vi "Teleop.vi"(10 "Match Info":T1={"Autonomous Elapsed Seconds"=0.0, "TeleOp Elapsed Seconds"=0.0, "Disabled Elapsed Seconds"=0.0, "Visited Autonomous"=FALSE, "Visited TeleOp"=FALSE, "Visited Disabled"=FALSE, "Autonomous Settings"={"Autonomous Style"=enum."Independent", "VI Refnum"=refnum}}, 11 "Call Context":T2) -> ()   [LabVIEW 2017]
doc: "This VI is called for each TeleOp packet received from the DS where the robot is not disabled. It is often used to read from the joysticks and update I/O or to update setpoints for timed control loops. It should complete and return within 20 milliseconds or it may miss DS packets."
uses:
  <vilib>/Rock Robotics/WPI/DriverStation/WPI_DriverStationDerivedRobotMode.ctl
  <vilib>/Rock Robotics/WPI/DriverStation/WPI_DriverStationMatch Info.ctl
  <vilib>/Rock Robotics/WPI/Utilities/WPI_GetSetVariantRefNum.vi
  <vilib>/Rock Robotics/Network Tables/NT Write Boolean Array.vi
  <vilib>/Rock Robotics/Network Tables/NT Write Numeric Array.vi
  <vilib>/Rock Robotics/Network Tables/NT Read Boolean.vi
  <vilib>/Rock Robotics/Network Tables/NT Read Number.vi
  <vilib>/Rock Robotics/WPI/RobotDrive/WPI_RobotDriveMecanumDrive_Cartesian.vi
panel:
  out "Numeric":dbl
  out "Sample Slider 0":dbl(slide) scale=0.0..5.0
  out "Sample Boolean 1":bool
  out "Sample Boolean 0":bool
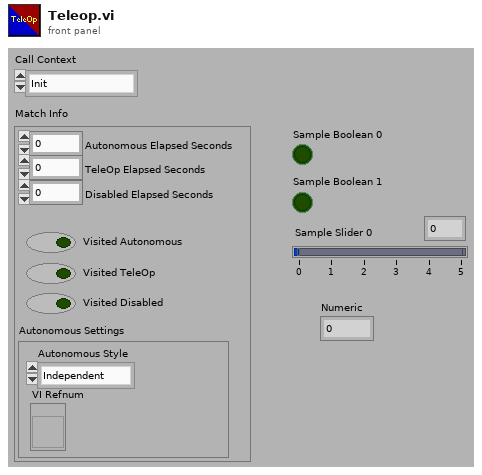
[diagram p1: front panel]
types:
  T1 = typedef "WPI_DriverStationMatch Info.ctl" = cluster{"Autonomous Elapsed Seconds":dbl, "TeleOp Elapsed Seconds":dbl, "Disabled Elapsed Seconds":dbl, "Visited Autonomous":bool, "Visited TeleOp":bool, "Visited Disabled":bool, "Autonomous Settings":cluster{"Autonomous Style":enum16{"Iterative", "Independent"}, "VI Refnum":refnum<vi>}}
  T2 = typedef "WPI_DriverStationDerivedRobotMode.ctl" = enum16{"Init", "Execute", "Stop"}
  T3 = typedef "WPI_JoystickDevRef.ctl" = cluster{"Device":T4}
  T4 = typedef "WPI_JoystickDeviceEnum.ctl" = enum16{"USB 0", "USB 1", "USB 2", "USB 3", "USB 4", "USB 5"}
  T5 = typedef "WPI_MotorControlDeviceRef.ctl" = cluster{"DeviceStatus":errorcluster, "Type":T6, "PWM":cluster{"PWM Channel":T7, "DeadBand":T8}, "CAN":cluster{"Device Number":u8, "SetOutput VI Ref":variant, "GetOutput VI Ref":variant, "Enable VI Ref":variant, "Disable VI Ref":variant, "Data":variant}, "Invert":bool, "DIO PWM":cluster{"PWM \"Enable\" Channel":T7, "DIOChannel":T9, "PWM Rate":dbl}}
  T6 = typedef "WPI_MotorControlType.ctl" = enum16{"PWM", "CAN", "DIO PWM"}
  T7 = typedef "FPGA_DIOPWMChannel.ctl" = enum8{"PWM 0", "PWM 1", "PWM 2", "PWM 3", "PWM 4", "PWM 5", "PWM 6", "PWM 7", "PWM 8", "PWM 9", "PWM MXP 0", "PWM MXP 1", "PWM MXP 2", "PWM MXP 3", "PWM MXP 4", "PWM MXP 5", "PWM MXP 6", "PWM MXP 7", "PWM MXP 8", "PWM MXP 9", "Invalid"}
  T8 = typedef "WPI_PWMDeadband.ctl" = cluster{"Name":string, "maxPositivePwm":i32, "minPositivePwm":i32, "centerPwm":i32, "maxNegativePwm":i32, "minNegativePwm":i32, "angularRange":u16}
  T9 = typedef "FPGA_DIOChannel.ctl" = enum8{"DIO 0", "DIO 1", "DIO 2", "DIO 3", "DIO 4", "DIO 5", "DIO 6", "DIO 7", "DIO 8", "DIO 9", "DIO MXP 0", "DIO MXP 1", "DIO MXP 2", "DIO MXP 3", "DIO MXP 4", "DIO MXP 5", "DIO MXP 6", "DIO MXP 7", "DIO MXP 8", "DIO MXP 9", "DIO MXP 10", "DIO MXP 11", "DIO MXP 12", "DIO MXP 13", "DIO MXP 14", "DIO MXP 15", "SPI Port CS1", "SPI Port CS2", "SPI Port CS3", "SPI Port MISO", "SPI Port MOSI", "Invalid"}
  T10 = typedef "WPI_RobotDriveDevRef.ctl" = cluster{"DevStatus":errorcluster, "Motors[]":T5[], "Square Inputs":bool, "Max Output":dbl}
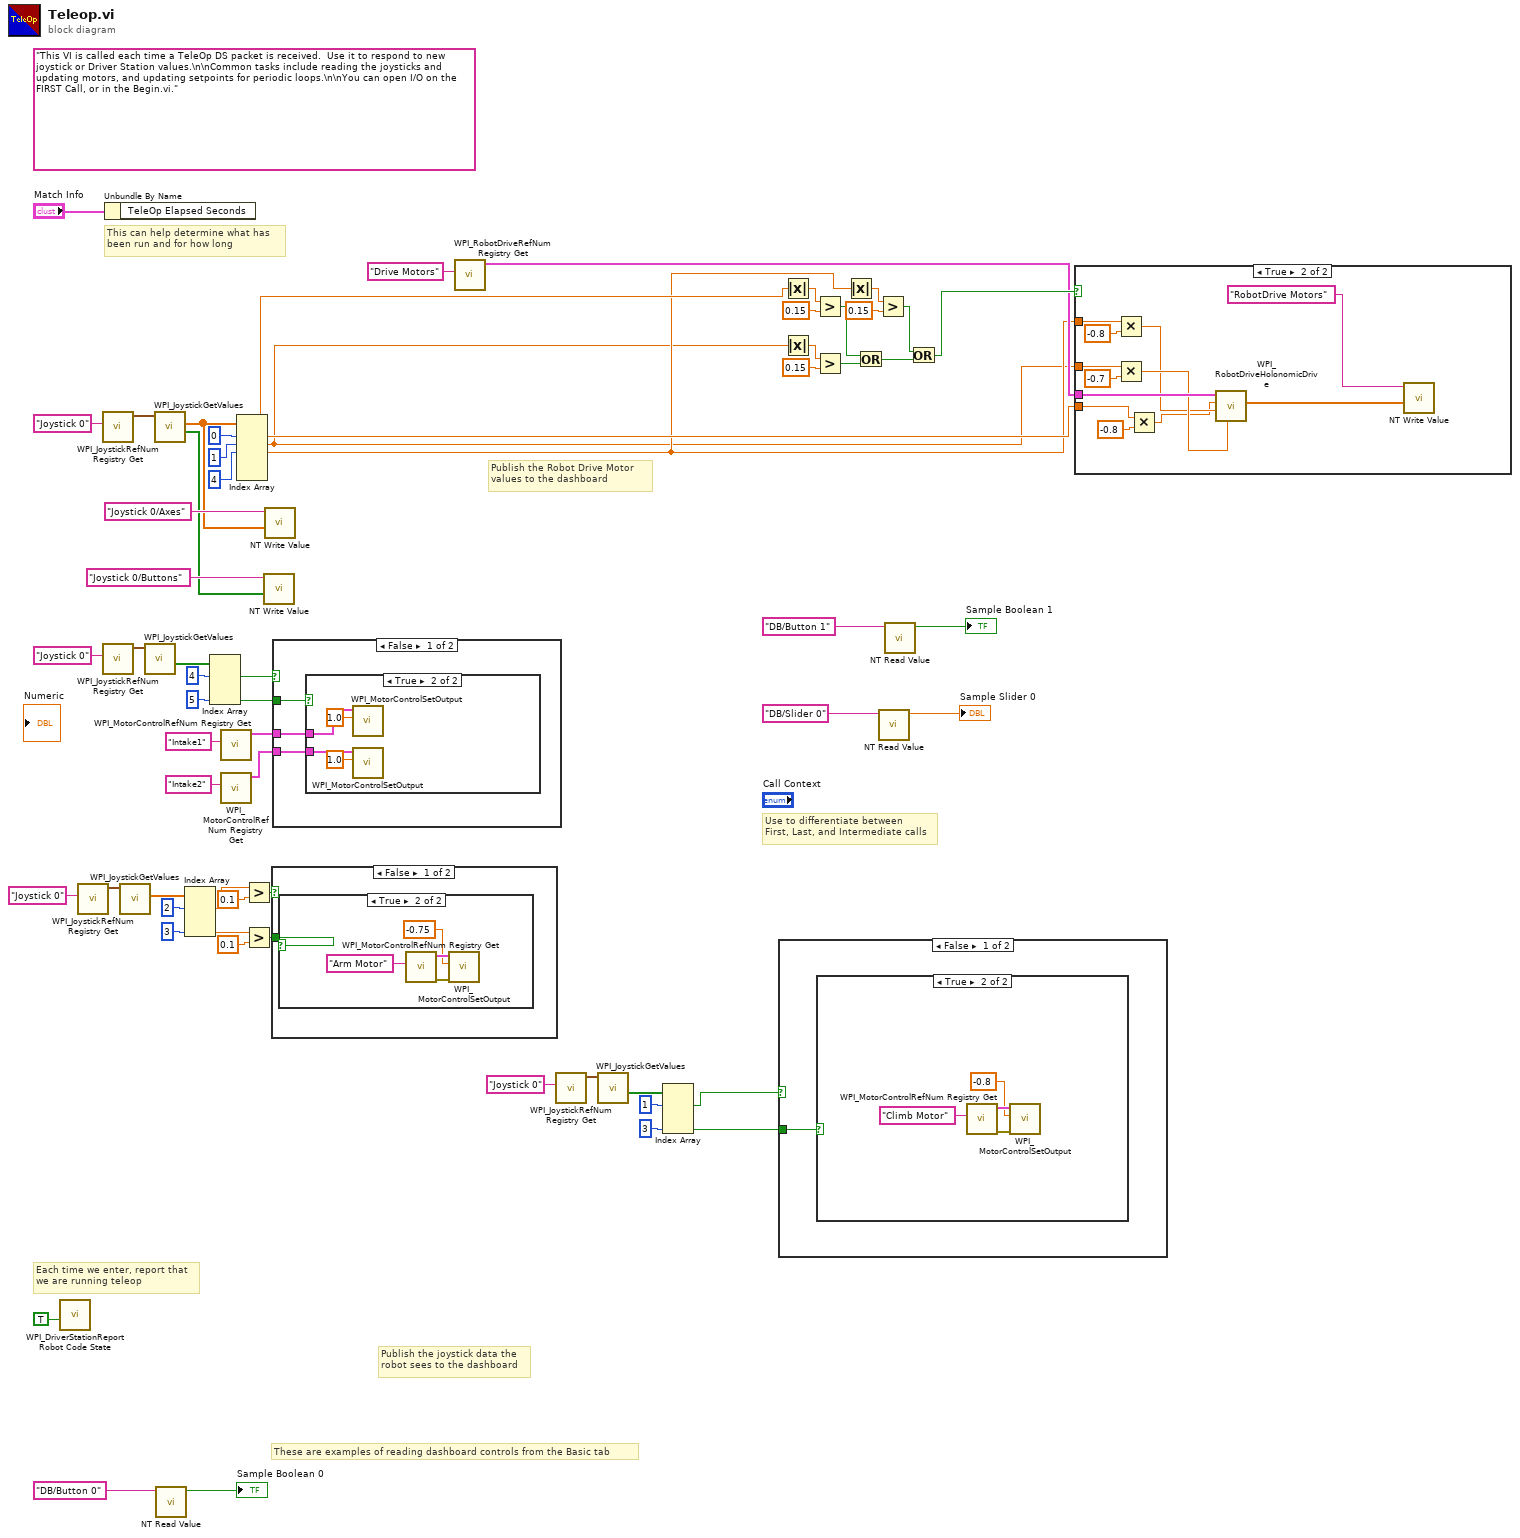
[diagram p0: block diagram]
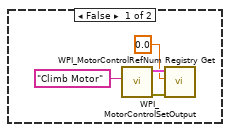
[diagram p3: hidden frame]
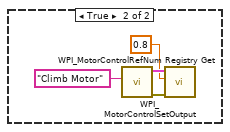
[diagram p4: hidden frame]
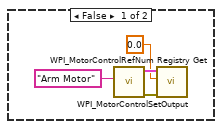
[diagram p5: hidden frame]
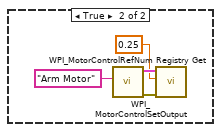
[diagram p6: hidden frame]
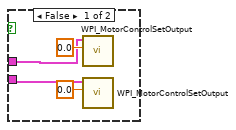
[diagram p7: hidden frame]
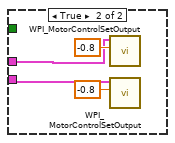
[diagram p8: hidden frame]
diagram:
  (unwired) "This VI is called each time a TeleOp DS packet is received.  Use it to respond to new joystick or Driver Station values.\n\nCommon tasks include reading the joysticks and updating motors, and updating setpoints for periodic loops.\n\nYou can open I/O on the FIRST Call, or in the Begin.vi."
  # "These are examples of reading dashboard controls from the Basic tab"
  # "Publish the Robot Drive Motor\nvalues to the dashboard"
  # "Publish the joystick data the\nrobot sees to the dashboard"
  # "Each time we enter, report that\nwe are running teleop"
  # "Use to differentiate between\nFirst, Last, and Intermediate calls"
  # "This can help determine what has\nbeen run and for how long"
  n1 = call <vilib>:"WPI_DriverStationReport Robot Code State.vi"("TeleOp"=TRUE ("Autonomous")) -> ()  [unwired: 10 in, 1 out]
  n2 = call <vilib>:"WPI_JoystickRefNum Registry Get.vi"("refnum name"="Joystick 0") -> ("JoystickDevRef"=w36:T3)  [unwired: 1 in, 9 out]
  n3 = call <vilib>:"WPI_JoystickRefNum Registry Get.vi"("refnum name"="Joystick 0") -> ("JoystickDevRef"=w59:T3)  [unwired: 1 in, 9 out]
  n4 = call <vilib>:"WPI_JoystickRefNum Registry Get.vi"("refnum name"="Joystick 0") -> ("JoystickDevRef"=w46:T3)  [unwired: 1 in, 9 out]
  n5 = Unbundle By Name("Match Info") -> ()  [unwired: 1 out]
  n6 = call <vilib>:"WPI_JoystickGetValues.vi"("JoystickDevRef"=w36) -> ("Axes"=w33:dbl[])  [unwired: 6 in, 4 out]
  n7 = call <vilib>:"WPI_JoystickGetValues.vi"("JoystickDevRef"=w46) -> ("Buttons"=w40:bool[])  [unwired: 6 in, 4 out]
  n8 = call <vilib>:"WPI_JoystickGetValues.vi"("JoystickDevRef"=w59) -> ("Buttons"=w54:bool[], "Axes"=w55:dbl[])  [unwired: 6 in, 3 out]
  n9 = call-poly <vilib>:"NT Read Value.vi"("Name"="DB/Button 0" ("refnum name")) -> ("Boolean"=→"Sample Boolean 0":bool)  [unwired: 9 in, 1 out]
  n10 = Index Array(array=w33, index #1=2 ("index"), index #4=3 ("index")) -> (element #1=w32:dbl, element #4=w29:dbl)  [unwired: 2 in, 2 out]
  n11 = Index Array(array=w40, index #1=4 ("index"), index #4=5 ("index")) -> (element #1=w39:bool, element #4=w38:bool)  [unwired: 2 in, 2 out]
  n12 = call <vilib>:"WPI_MotorControlRefNum Registry Get.vi"("refnum name"="Intake1") -> ("MotorControlDevRef"=w1:T5)  [unwired: 9 in, 1 out]
  n13 = call <vilib>:"WPI_MotorControlRefNum Registry Get.vi"("refnum name"="Intake2") -> ("MotorControlDevRef"=w2:T5)  [unwired: 9 in, 1 out]
  n14 = Index Array(array=w55, index #1=0 ("index"), index #2=1 ("index"), index #3=4 ("index")) -> (element #1=w10:dbl, element #2=w6:dbl, element #3=w8:dbl)  [unwired: 3 in, 3 out]
  n15 = Greater?(x=w32, y=0.1) -> (0:w30:bool)
  n16 = Greater?(x=w29, y=0.1) -> (0:w20:bool)
  n17 = call-poly <vilib>:"NT Write Value.vi"("Boolean Array"=w54, "Name"="Joystick 0/Buttons") -> ()  [unwired: 9 in, 1 out]
  n18 = call-poly <vilib>:"NT Write Value.vi"("Numeric Array"=w55, "Name"="Joystick 0/Axes") -> ()  [unwired: 9 in, 1 out]
  n19 = case shown="False" w30 {
    tunnel: w20 -> [w63 _]
    frame False {
      n20 = case shown="True" w63 {
        frame False {
          n21 = call <vilib>:"WPI_MotorControlRefNum Registry Get.vi"("refnum name"="Arm Motor") -> ("error out"=w67:errorcluster, "MotorControlDevRef"=w66:T5)  [unwired: 9 in]
          n22 = call <vilib>:"WPI_MotorControlSetOutput.vi"("error in (no error)"=w67, "Output"=0.0, "MotorControlDevRef"=w66) -> ()  [unwired: 6 in, 3 out]
        }
        frame True {
          n23 = call <vilib>:"WPI_MotorControlRefNum Registry Get.vi"("refnum name"="Arm Motor") -> ("error out"=w71:errorcluster, "MotorControlDevRef"=w70:T5)  [unwired: 9 in]
          n24 = call <vilib>:"WPI_MotorControlSetOutput.vi"("error in (no error)"=w71, "Output"=-0.75, "MotorControlDevRef"=w70) -> ()  [unwired: 6 in, 3 out]
        }
      }
    }
    frame True {
      n25 = call <vilib>:"WPI_MotorControlRefNum Registry Get.vi"("refnum name"="Arm Motor") -> ("error out"=w75:errorcluster, "MotorControlDevRef"=w74:T5)  [unwired: 9 in]
      n26 = call <vilib>:"WPI_MotorControlSetOutput.vi"("error in (no error)"=w75, "Output"=0.25, "MotorControlDevRef"=w74) -> ()  [unwired: 6 in, 3 out]
    }
  }
  n27 = case shown="False" w39 {
    tunnel: w38 -> [w78 _]
    tunnel: w2 -> [w77 w87]
    tunnel: w1 -> [w76 w88]
    frame False {
      n28 = case shown="True" w78 {
        tunnel: w77 -> [w79 w86]
        tunnel: w76 -> [w80 w85]
        frame False {
          n29 = call <vilib>:"WPI_MotorControlSetOutput.vi"("Output"=0.0, "MotorControlDevRef"=w80) -> ()  [unwired: 7 in, 3 out]
          n30 = call <vilib>:"WPI_MotorControlSetOutput.vi"("Output"=0.0, "MotorControlDevRef"=w79) -> ()  [unwired: 7 in, 3 out]
        }
        frame True {
          n31 = call <vilib>:"WPI_MotorControlSetOutput.vi"("Output"=1.0, "MotorControlDevRef"=w85) -> ()  [unwired: 7 in, 3 out]
          n32 = call <vilib>:"WPI_MotorControlSetOutput.vi"("Output"=1.0, "MotorControlDevRef"=w86) -> ()  [unwired: 7 in, 3 out]
        }
      }
    }
    frame True {
      n33 = call <vilib>:"WPI_MotorControlSetOutput.vi"("Output"=-0.8, "MotorControlDevRef"=w88) -> ()  [unwired: 7 in, 3 out]
      n34 = call <vilib>:"WPI_MotorControlSetOutput.vi"("Output"=-0.8, "MotorControlDevRef"=w87) -> ()  [unwired: 7 in, 3 out]
    }
  }
  n35 = call <vilib>:"WPI_RobotDriveRefNum Registry Get.vi"("refnum name"="Drive Motors") -> ("RobotDriveDevRef"=w11:T10)  [unwired: 1 in, 9 out]
  n36 = call <vilib>:"WPI_JoystickRefNum Registry Get.vi"("refnum name"="Joystick 0") -> ("JoystickDevRef"=w26:T3)  [unwired: 1 in, 9 out]
  n37 = call <vilib>:"WPI_JoystickGetValues.vi"("JoystickDevRef"=w26) -> ("Buttons"=w23:bool[])  [unwired: 6 in, 4 out]
  n38 = Index Array(array=w23, index #1=1 ("index"), index #4=3 ("index")) -> (element #1=w22:bool, element #4=w21:bool)  [unwired: 2 in, 2 out]
  n39 = case shown="False" w22 {
    tunnel: w21 -> [w91 _]
    frame False {
      n40 = case shown="True" w91 {
        frame False {
          n41 = call <vilib>:"WPI_MotorControlRefNum Registry Get.vi"("refnum name"="Climb Motor") -> ("error out"=w95:errorcluster, "MotorControlDevRef"=w94:T5)  [unwired: 9 in]
          n42 = call <vilib>:"WPI_MotorControlSetOutput.vi"("error in (no error)"=w95, "Output"=0.0, "MotorControlDevRef"=w94) -> ()  [unwired: 6 in, 3 out]
        }
        frame True {
          n43 = call <vilib>:"WPI_MotorControlRefNum Registry Get.vi"("refnum name"="Climb Motor") -> ("error out"=w99:errorcluster, "MotorControlDevRef"=w98:T5)  [unwired: 9 in]
          n44 = call <vilib>:"WPI_MotorControlSetOutput.vi"("error in (no error)"=w99, "Output"=-0.8, "MotorControlDevRef"=w98) -> ()  [unwired: 6 in, 3 out]
        }
      }
    }
    frame True {
      n45 = call <vilib>:"WPI_MotorControlRefNum Registry Get.vi"("refnum name"="Climb Motor") -> ("error out"=w103:errorcluster, "MotorControlDevRef"=w102:T5)  [unwired: 9 in]
      n46 = call <vilib>:"WPI_MotorControlSetOutput.vi"("error in (no error)"=w103, "Output"=0.8, "MotorControlDevRef"=w102) -> ()  [unwired: 6 in, 3 out]
    }
  }
  n47 = Absolute Value(x=w10) -> (abs(x)=w9:dbl)
  n48 = Absolute Value(x=w6) -> (abs(x)=w5:dbl)
  n49 = Greater?(x=w9, y=0.15) -> (0:w14:bool)
  n50 = Greater?(x=w5, y=0.15) -> (0:w13:bool)
  n51 = Absolute Value(x=w8) -> (abs(x)=w7:dbl)
  n52 = Or(x=w14, y=w13) -> (x .or. y?=w19:bool)
  n53 = Greater?(x=w7, y=0.15) -> (0:w15:bool)
  n54 = call-poly <vilib>:"NT Read Value.vi"("Name"="DB/Slider 0" ("refnum name")) -> ("Numeric"=→"Sample Slider 0":dbl)  [unwired: 9 in, 1 out]
  n55 = call-poly <vilib>:"NT Read Value.vi"("Name"="DB/Button 1" ("refnum name")) -> ("Boolean"=→"Sample Boolean 1":bool)  [unwired: 9 in, 1 out]
  n56 = Or(x=w15, y=w19) -> (x .or. y?=w12:bool)
  n57 = case shown="True" w12 {
    tunnel: w6 -> [_ w111]
    tunnel: w8 -> [_ w108]
    tunnel: w10 -> [_ w104]
    tunnel: w11 -> [_ w114]
    frame False {
    }
    frame True {
      n58 = Multiply(x=w108, y=-0.8) -> (x*y=w107:dbl)
      n59 = Multiply(x=w111, y=-0.7) -> (x*y=w110:dbl)
      n60 = Multiply(x=w104, y=-0.8) -> (x*y=w105:dbl)
      n61 = call-poly <vilib>:"WPI_RobotDriveHolonomicDrive.vi"("Rotation"=w110, "Y"=w107, "X"=w105, "RobotDriveDevRef"=w114) -> ("Motor Values"=w115:dbl[])  [unwired: 5 in, 2 out]
      n62 = call-poly <vilib>:"NT Write Value.vi"("Numeric Array"=w115, "Name"="RobotDrive Motors") -> ()  [unwired: 9 in, 1 out]
    }
  }
